vi "Read azElTracking.vi"(8 "error in (no error)":errorcluster, 11 "TCSMccStatus in":refnum<class "TCSMccStatus.lvclass">) -> (0 "error out":errorcluster, 2 "AzElTracking.lvclass":refnum<class "AzElTracking.lvclass">, 3 "TCSMccStatus out":refnum<class "TCSMccStatus.lvclass">)   [LabVIEW 2014, in "TCSDataDefinitions.lvlib" / "TCSMountControlStatus.lvlib" / "TCSMccStatus.lvclass"]
uses:
  TCSMccStatus.lvclass
  AzElTracking/AzElTracking/AzElTracking.lvclass
  TCSMccStatus.lvclass/TCSMccStatus.ctl
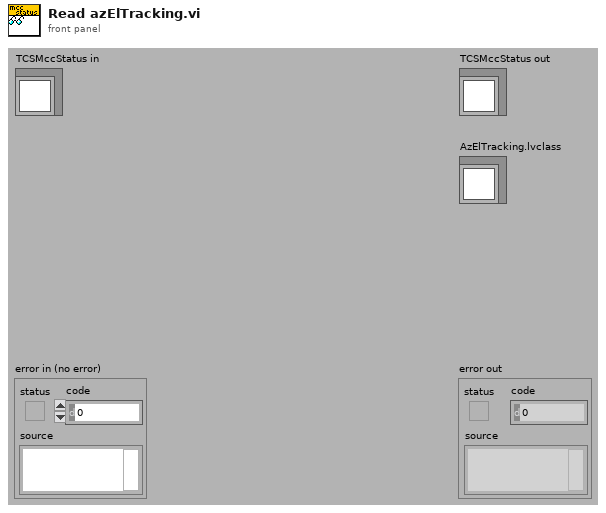
[diagram p1: front panel]
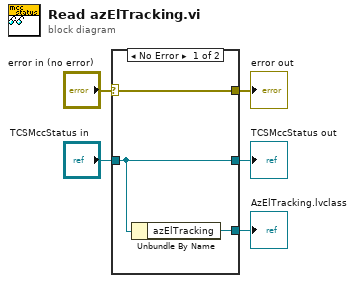
[diagram p0: block diagram]
diagram:
  n1 = case shown="No Error" "error in (no error)" {
    selector: "error in (no error)" -> [w8 w9]
    tunnel: [w8 w9] -> w4
    tunnel: [w7 w10] -> w2
    tunnel: "TCSMccStatus in" -> [w7 w10]
    tunnel: [w6 _] -> w1
    frame No Error {
      n2 = Unbundle By Name(w7) -> ("azElTracking"=w6:refnum<class "AzElTracking.lvclass">)
    }
    frame Error {
    }
  }
  "error out" <- w4
  "TCSMccStatus out" <- w2
  "AzElTracking.lvclass" <- w1
